vi "RiversideRelaySetChannel.vi"(0 "serial_number":string="Z8KHE", 1 "Transducer":enum16{"Transducer 1", "Transducer 2"}(ring), 2 "Relay Channel":i32=1, 3 "error in":errorcluster) -> (5 "Active Relay Channel":i32=1, 6 "Change Polarity":i32, 7 "error out":errorcluster)   [LabVIEW 2022 SP3]
uses:
  SwitchGlobals.vi
  usb_relay_device/usb_relay_device.lvlib
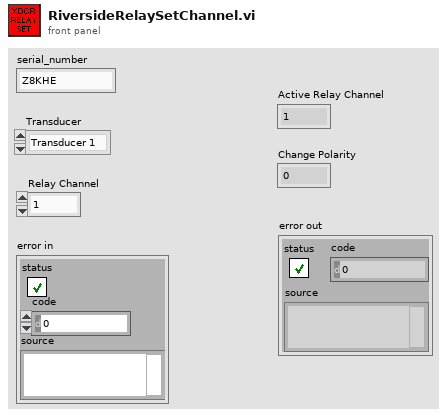
[diagram p1: front panel]
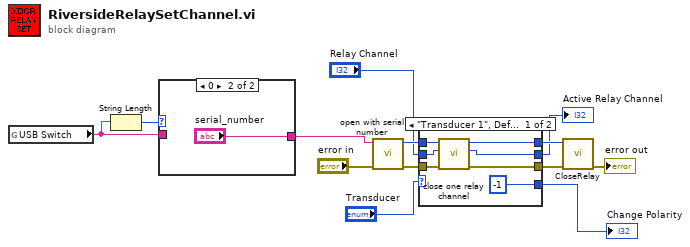
[diagram p0: block diagram]
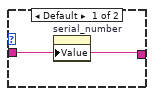
[diagram p2: hidden frame]
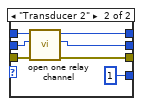
[diagram p3: hidden frame]
diagram:
  n1 = global read "SwitchGlobals.vi" "USB Switch"() -> (w1:string)
  n2 = String Length(string=w1) -> (length=w2:i32)
  n3 = case shown="0" w2 {
    tunnel: [w14 "serial_number"] -> w13
    tunnel: w1 -> [w14 _]
    frame Default {
      n4 = property on="serial_number" class="Str"("Value"=w14) -> ()  [unwired: 2 in, 2 out]
    }
    frame 0 {
    }
  }
  n5 = call "open with serial number.vi"("error in (no error)"="error in", "serial_number"=w13) -> ("error out"=w11:errorcluster, "Relay Identifier"=w12:i32)  [unwired: 8 in]
  n6 = case shown="\"Transducer 1\", Default" "Transducer" {
    tunnel: w12 -> [w17 w29]
    tunnel: w11 -> [w19 w28]
    tunnel: [w22 w27] -> w10
    tunnel: [w20 w26] -> w9
    tunnel: "Relay Channel" -> [w18 w25]
    tunnel: [w21 w24] -> w7
    tunnel: [-1 1] -> w3
    frame "Transducer 1", Default {
      n7 = call "close one relay channel.vi"("error in (no error)"=w19, "Relay Channel"=w18, "Relay Identifier"=w17) -> ("error out"=w20:errorcluster, "Closed Relay Channel"=w21:i32, "Relay Indetifier Out"=w22:i32)  [unwired: 6 in]
    }
    frame "Transducer 2" {
      n8 = call "open one relay channel.vi"("error in (no error)"=w28, "Relay Channel"=w25, "Relay Identifier"=w29) -> ("error out"=w26:errorcluster, "Active Relay Channel"=w24:i32, "Relay Indetifier Out"=w27:i32)  [unwired: 6 in]
    }
  }
  "Active Relay Channel" <- w7
  "Change Polarity" <- w3
  n9 = call "CloseRelay.vi"("error in (no error)"=w9, "Relay Identifier"=w10) -> ("error out"=→"error out":errorcluster)  [unwired: 9 in]
